vi "WPI_RobotDriveSafetyError.vi"(0 "RobotDriveDevRef":T1={"DevStatus"={"status"=FALSE, "code"=0, "source"=""}, "Motors[]"=[], "Square Inputs"=FALSE, "Max Output"=1.0}) -> ()   [LabVIEW 2017]
doc: "This subVI does two things:\n1. It builds up output specific information to help locate the problem.\n2. It calls the FRC Build Error, so all the information gets passed to the Driver Station."
uses:
  <vilib>/Rock Robotics/WPI/RobotDrive/WPI_RobotDriveDevRef.ctl
  <vilib>/Rock Robotics/WPI/MotorControl/WPI_MotorControlDeviceRef.ctl
  <vilib>/Rock Robotics/WPI/MotorControl/WPI_MotorControlType.ctl
  <vilib>/Rock Robotics/SystemInterfaces/DIO/FPGA_DIOPWMChannel.ctl
  <vilib>/Rock Robotics/WPI/PWM/WPI_PWMDeadband.ctl
  <vilib>/Rock Robotics/SystemInterfaces/DIO/FPGA_DIOChannel.ctl
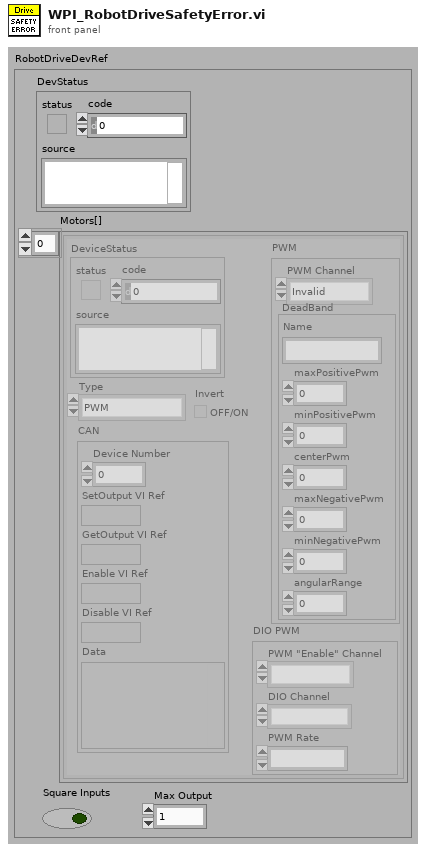
[diagram p1: front panel]
types:
  T1 = typedef "WPI_RobotDriveDevRef.ctl" = cluster{"DevStatus":errorcluster, "Motors[]":T2[], "Square Inputs":bool, "Max Output":dbl}
  T2 = typedef "WPI_MotorControlDeviceRef.ctl" = cluster{"DeviceStatus":errorcluster, "Type":T3, "PWM":cluster{"PWM Channel":T4, "DeadBand":T5}, "CAN":cluster{"Device Number":u8, "SetOutput VI Ref":variant, "GetOutput VI Ref":variant, "Enable VI Ref":variant, "Disable VI Ref":variant, "Data":variant}, "Invert":bool, "DIO PWM":cluster{"PWM \"Enable\" Channel":T4, "DIOChannel":T6, "PWM Rate":dbl}}
  T3 = typedef "WPI_MotorControlType.ctl" = enum16{"PWM", "CAN", "DIO PWM"}
  T4 = typedef "FPGA_DIOPWMChannel.ctl" = enum8{"PWM 0", "PWM 1", "PWM 2", "PWM 3", "PWM 4", "PWM 5", "PWM 6", "PWM 7", "PWM 8", "PWM 9", "PWM MXP 0", "PWM MXP 1", "PWM MXP 2", "PWM MXP 3", "PWM MXP 4", "PWM MXP 5", "PWM MXP 6", "PWM MXP 7", "PWM MXP 8", "PWM MXP 9", "Invalid"}
  T5 = typedef "WPI_PWMDeadband.ctl" = cluster{"Name":string, "maxPositivePwm":i32, "minPositivePwm":i32, "centerPwm":i32, "maxNegativePwm":i32, "minNegativePwm":i32, "angularRange":u16}
  T6 = typedef "FPGA_DIOChannel.ctl" = enum8{"DIO 0", "DIO 1", "DIO 2", "DIO 3", "DIO 4", "DIO 5", "DIO 6", "DIO 7", "DIO 8", "DIO 9", "DIO MXP 0", "DIO MXP 1", "DIO MXP 2", "DIO MXP 3", "DIO MXP 4", "DIO MXP 5", "DIO MXP 6", "DIO MXP 7", "DIO MXP 8", "DIO MXP 9", "DIO MXP 10", "DIO MXP 11", "DIO MXP 12", "DIO MXP 13", "DIO MXP 14", "DIO MXP 15", "SPI Port CS1", "SPI Port CS2", "SPI Port CS3", "SPI Port MISO", "SPI Port MOSI", "Invalid"}
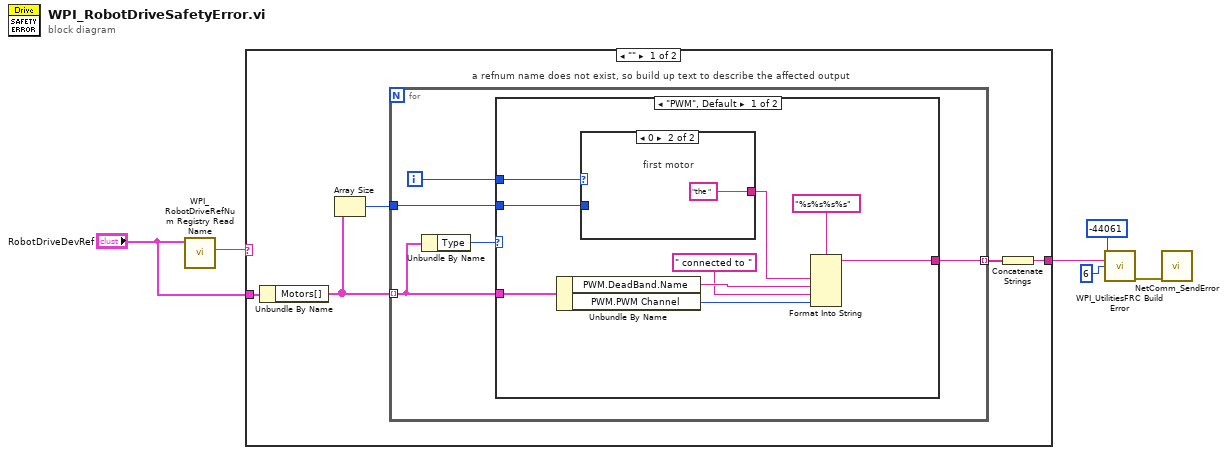
[diagram p0: block diagram]
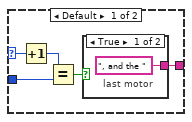
[diagram p2: hidden frame]
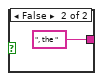
[diagram p3: hidden frame]
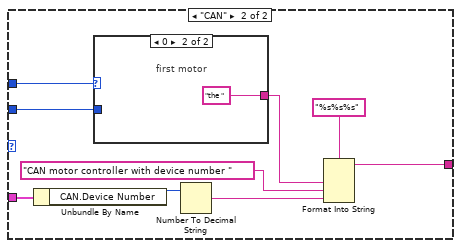
[diagram p4: hidden frame]
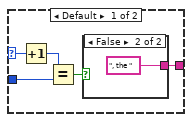
[diagram p5: hidden frame]
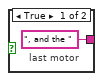
[diagram p6: hidden frame]
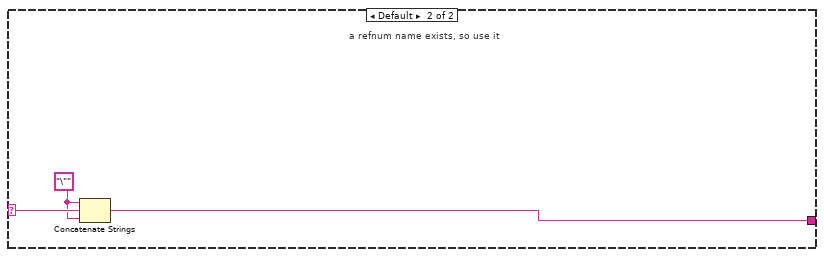
[diagram p7: hidden frame]
diagram:
  n1 = call <vilib>:"WPI_RobotDriveRefNum Registry Read Name.vi"("RobotDriveDevRef"="RobotDriveDevRef") -> ("refnum name"=w3:string)  [unwired: 1 in, 9 out]
  n2 = case shown="\"\"" w3 {
    selector: w3 -> [_ w53]
    tunnel: [w7 w52] -> w2
    tunnel: "RobotDriveDevRef" -> [w11 _]
    frame "" {
      # "a refnum name does not exist, so build up text to describe the affected output"
      n3 = Unbundle By Name(w11) -> ("Motors[]"=w9:T2[])
      n4 = Array Size(array=w9) -> (size(s)=w8:i32)
      n5 = for {
        tunnel: w9 -> [w13] mode=indexing
        tunnel: [w16] -> w10 mode=indexing
        tunnel: w8 -> [w14]
        i -> [w15]
        n6 = Unbundle By Name(w13) -> ("Type"=w12:T3)
        n7 = case shown="\"PWM\", Default" w12 {
          tunnel: [w21 w41] -> w16
          tunnel: w15 -> [w20 w40]
          tunnel: w14 -> [w19 w39]
          tunnel: w13 -> [w17 w37]
          frame "PWM", Default {
            n8 = Unbundle By Name(w17) -> ("PWM.DeadBand.Name"=w24:string, "PWM.PWM Channel"=w22:T4)
            n9 = case shown="0" w20 {
              selector: w20 -> [w30 _]
              tunnel: w19 -> [w27 _]
              tunnel: [w26 "the " ("format string")] -> w18
              frame Default {
                n10 = Increment(x=w30) -> (x+1=w28:i32)
                n11 = Equal?(x=w28, y=w27) -> (x = y?=w29:bool)
                n12 = case shown="True" w29 {
                  tunnel: [", and the " ("format string") ", the " ("format string")] -> w26
                  frame True {
                    # "last motor"
                  }
                  frame False {
                  }
                }
              }
              frame 0 {
                # "first motor"
              }
            }
            n13 = Format Into String(format string="%s%s%s%s", w18, w24, " connected to " ("format string"), w22) -> (resulting string=w21:string)  [unwired: 2 in, 1 out]
          }
          frame "CAN" {
            n14 = Unbundle By Name(w37) -> ("CAN.Device Number"=w35:u8)
            n15 = case shown="0" w40 {
              selector: w40 -> [w47 _]
              tunnel: w39 -> [w44 _]
              tunnel: [w43 "the " ("format string")] -> w38
              frame Default {
                n16 = Increment(x=w47) -> (x+1=w45:i32)
                n17 = Equal?(x=w45, y=w44) -> (x = y?=w46:bool)
                n18 = case shown="False" w46 {
                  tunnel: [", and the " ("format string") ", the " ("format string")] -> w43
                  frame True {
                    # "last motor"
                  }
                  frame False {
                  }
                }
              }
              frame 0 {
                # "first motor"
              }
            }
            n19 = Number To Decimal String(number=w35) -> (decimal integer string=w36:string)  [unwired: 1 out]
            n20 = Format Into String(format string="%s%s%s", w38, "CAN motor controller with device number " ("format string"), w36) -> (resulting string=w41:string)  [unwired: 2 in, 1 out]
          }
        }
      }
      n21 = Concatenate Strings(w10) -> (w7:string)
    }
    frame Default {
      w51 = "\"" ("string")
      # "a refnum name exists, so use it"
      n22 = Concatenate Strings(w51, w53, w51) -> (w52:string)
    }
  }
  n23 = call <vilib>:"WPI_UtilitiesFRC Build Error.vi"("error code"=-44061 ("code"), "extra error text"=w2, "chain levels to remove (1)"=6) -> ("error out"=w1:errorcluster)  [unwired: 3 in, 9 out]
  n24 = call <vilib>:"NetComm_SendError.vi"("error in (no error)"=w1) -> ()  [unwired: 11 in]
